vi "HVpulser_Wrapper.vi"(0 "Path Array":string[](array[string])=["C:\\CuspControl\\GPIB and Network\\HVpulser.txt", "6723"], 1 "Input Values":dbl[](array[numeric])=[0.0]) -> ()   [LabVIEW 2018]
uses:
  <vilib>/DAQmx/write.llb/DAQmx Write (Analog 1D DBL NChan 1Samp).vi
  <vilib>/DAQmx/create/channels.llb/DAQmx Create Channel (AO-Voltage-Basic).vi
  <vilib>/DAQmx/miscellaneous.llb/DAQmx Fill In Error Info.vi
panel:
  in  "# devices":i32=2
  in  "subvi":bool=TRUE
  in  "Default LV (10 V)":dbl=10.0
  in  "Gain (160 V/V)":dbl=160.0 format="%#_13g"
  in  "Max HV (V)":dbl=110.0
  out "LV (10 V)":dbl
  out "HV (/160 V)":dbl
  out "Time (s)":dbl=0.0015946000348776579
  out "Device names":string[](array[string])=["Dev5/ao6", "Dev5/ao7"]
  out "Set Values":dbl[](array[numeric])
  out "error out":errorcluster
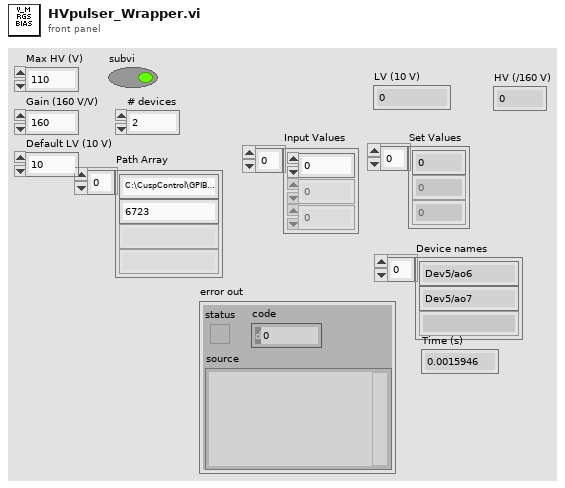
[diagram p1: front panel]
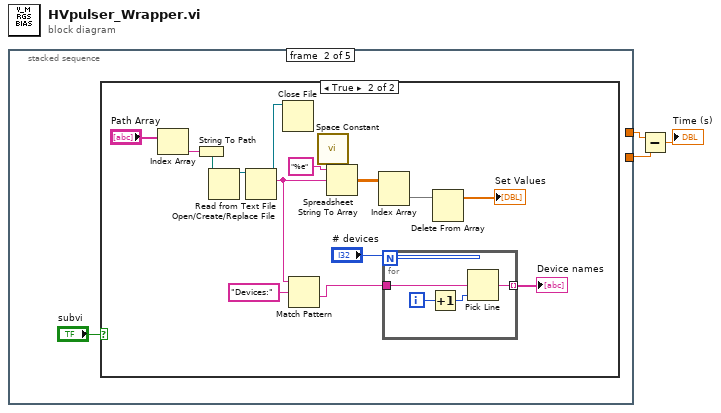
[diagram p0: block diagram]
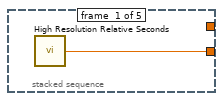
[diagram p2: hidden frame]
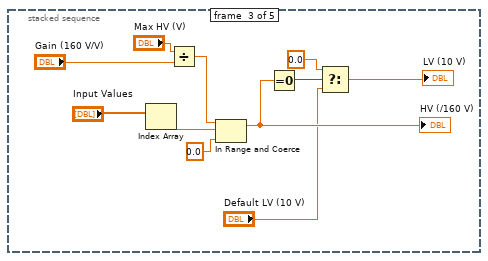
[diagram p4: hidden frame]
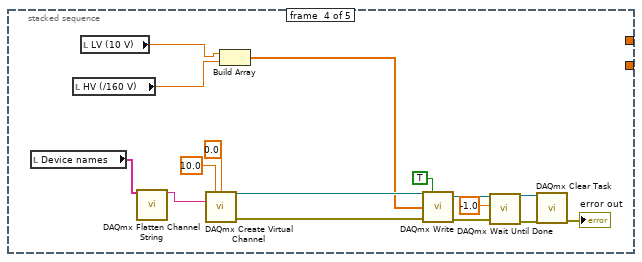
[diagram p5: hidden frame]
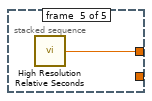
[diagram p6: hidden frame]
diagram:
  n1 = stacked-sequence {
    tunnel: [w4 _ _ _ _] -> w2
    tunnel: [_ _ _ _ w52] -> w3
    frame #0 {
      n2 = call <vilib>:"High Resolution Relative Seconds.vi"() -> ("relative seconds"=w4:dbl)
    }
    frame #1 {
      n3 = case shown="True" "subvi" {
        frame False {
        }
        frame True {
          n4 = Index Array(array="Path Array") -> (element=w19:string)  [unwired: 1 in]
          n5 = String To Path(string=w19) -> (path=w7:path)
          n6 = Open/Create/Replace File(file path (use dialog)=w7) -> (refnum out=w9:refnum<file>)  [unwired: 5 in, 2 out]
          n7 = Read from Text File(file (use dialog)=w9) -> (refnum out=w6:refnum<file>, text=w15:string)  [unwired: 3 in, 2 out]
          n8 = Close File(refnum=w6) -> ()  [unwired: 1 in, 2 out]
          n9 = Match Pattern(string=w15, regular expression="Devices:") -> (after substring=w13:string)  [unwired: 1 in, 3 out]
          n10 = call <vilib>:"Space Constant.vi"() -> ("String"=w17:string)
          n11 = Spreadsheet String To Array(delimiter (Tab)=w17, format string="%e", spreadsheet string=w15) -> (array=w16:dbl[][])  [unwired: 1 in]
          n12 = Index Array(array=w16) -> (element=w10:dbl[])  [unwired: 2 in]
          n13 = for {
            N: "# devices" -> [_]
            tunnel: w13 -> [w22]
            tunnel: [w21] -> w11 mode=indexing
            i -> [w24]
            n14 = Increment(x=w24) -> (x+1=w23:i32)
            n15 = Pick Line(multi-line string=w22, line index=w23) -> (output string=w21:string)  [unwired: 1 in]
          }
          "Device names" <- w11
          n16 = Delete From Array(array=w10) -> (array with subset deleted=→"Set Values":dbl[])  [unwired: 2 in, 1 out]
        }
      }
    }
    frame #2 {
      n17 = Index Array(array="Input Values") -> (element=w34:dbl)  [unwired: 1 in]
      n18 = Divide(x="Max HV (V)", y="Gain (160 V/V)") -> (x/y=w30:dbl)
      n19 = In Range and Coerce(upper limit=w30, x=w34, lower limit=0.0) -> (coerced(x)=w29:dbl)  [unwired: 1 out]
      "HV (/160 V)" <- w29
      n20 = Equal To 0?(x=w29) -> (x = 0?=w28:bool)
      n21 = Select(t=0.0, s=w28, f="Default LV (10 V)") -> (s? t:f=→"LV (10 V)":dbl)
    }
    frame #3 {
      n22 = local read "Device names"() -> (w42:string[])
      n23 = local read "HV (/160 V)"() -> (w38:dbl)
      n24 = local read "LV (10 V)"() -> (w36:dbl)
      n25 = call <vilib>:"DAQmx Flatten Channel String.vi"("names in"=w42) -> ("names out"=w41:string)  [unwired: 13 in, 1 out]
      n26 = call-poly <vilib>:"DAQmx Create Virtual Channel.vi"("maximum value"=10.0, "minimum value"=0.0, "physical channels"=w41) -> ("task out"=w40:refnum<k21>, "error out"=w39:errorcluster)  [unwired: 11 in]
      n27 = Build Array(w36, w38) -> (w37:dbl[])
      n28 = call-poly <vilib>:"DAQmx Write.vi"("task/channels in"=w40, "auto start"=TRUE, "data"=w37, "error in"=w39) -> ("task out"=w45:refnum<k21>, "error out"=w44:errorcluster)  [unwired: 9 in, 1 out]
      n29 = call <vilib>:"DAQmx Wait Until Done.vi"("task/channels in"=w45, "timeout (sec)"=-1.0, "error in"=w44) -> ("task out"=w46:refnum<k21>, "error out"=w47:errorcluster)  [unwired: 11 in]
      n30 = call <vilib>:"DAQmx Clear Task.vi"("task in"=w46, "error in"=w47) -> ("error out"=→"error out":errorcluster)  [unwired: 13 in]
    }
    frame #4 {
      n31 = call <vilib>:"High Resolution Relative Seconds.vi"() -> ("relative seconds"=w52:dbl)
    }
  }
  n32 = Subtract(x=w3, y=w2) -> (x-y=→"Time (s)":dbl)
